vi "Update Entity.vi"(7 "Project Ref":refnum<vi>, 8 "error in (no error)":errorcluster, 9 "Definition":T1[](array[typedef]), 10 "Entity Path":path, 11 "Entity Editor in":refnum<class "Entity Editor.lvclass">) -> (0 "error out":errorcluster, 3 "Entity Editor out":refnum<class "Entity Editor.lvclass">)   [LabVIEW 2020, in "Conditum-Tools.lvlib" / "Entity Editor.lvclass"]
uses:
  Entity Editor.lvclass
  Field Config.ctl
  Conditum-Clone/Columns/Type/Type.lvclass
  Accessors.ctl
  Accessor Scope.ctl
  Entity Editor.lvclass/Entity Editor.ctl
  1745b105-25e8-435b-8540-0ac186d7c8ff.vi
  6bb5155e-7406-4f3e-8756-88858d5c17d7.vi
  Update Entity OoC.vi
  Editor Context.vi
  Conditum-Tools.lvlib
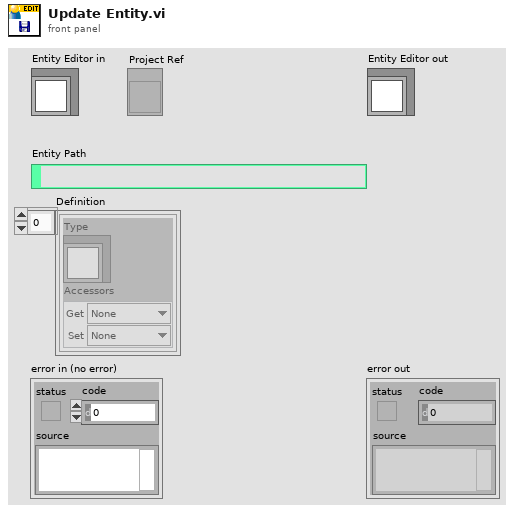
[diagram p1: front panel]
types:
  T1 = typedef "Conditum-Tools.lvlib/Field Config.ctl" = cluster{"Type":refnum<class "Type.lvclass">, "Accessors":T2}
  T2 = typedef "Conditum-Tools.lvlib/Accessors.ctl" = cluster{"Get":T3, "Set":T3}
  T3 = typedef "Conditum-Tools.lvlib/Accessor Scope.ctl" = enum16{"None", "Public", "Protected", "Private"}
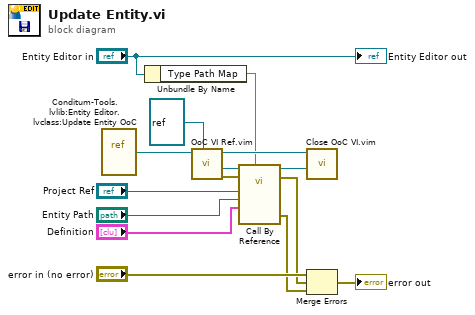
[diagram p0: block diagram]
diagram:
  n1 = vi-ref "Conditum-Tools.lvlib:Entity Editor.lvclass:Update Entity OoC.vi"() -> (w6:refnum<vi>)
  n2 = Unbundle By Name("Entity Editor in") -> ("Type Path Map"=w4:map{path, path})
  n3 = call "OoC VI Ref.vim"("VI Type"=refnum<vi> refnum, "OoC SVR"=w6) -> ("error out"=w9:errorcluster, "vi reference"=w10:refnum<vi>, "context"=w8:refnum<vi>)  [unwired: 7 in]
  n4 = call-by-ref "?"(reference=w10, error in=w9, "Type Path Map"=w4, "Definition"="Definition", "Entity Path"="Entity Path", "Project Ref"="Project Ref") -> (reference out=w7:refnum<vi>, error out=w12:errorcluster, 0:"error out"=w11:errorcluster)  [unwired: 7 in]
  n5 = call "Close OoC VI.vim"("vi reference"=w7, "context"=w8) -> ()  [unwired: 9 in, 1 out]
  n6 = Merge Errors("error in (no error)", w12, w11) -> (→"error out":errorcluster)
  "Entity Editor out" <- "Entity Editor in"
